vi "updateBall.vi"(8 "error in (no error)":errorcluster, 10 "old Ball":refnum<class "Ball.lvclass">, 11 "Ball in":refnum<class "Ball.lvclass">) -> (0 "error out":errorcluster, 3 "Ball out":refnum<class "Ball.lvclass">)   [LabVIEW 2020, in "Ball.lvclass"]
uses:
  Ball.lvclass
  C:/Users/Administrator/Desktop/SSL/SSL_AI/Object_class/Object.lvclass
  Object_class/Object.lvclass/Object.ctl
  Ball.lvclass/Ball.ctl
  Object_class/Read x.vi
  Object_class/Read y.vi
  Read v_x.vi
  Read v_y.vi
  Object_class/Read pos_est_x.vi
  Object_class/Read pos_est_y.vi
  Read Valid.vi
  Read z.vi
  Object_class/Write x.vi
  Object_class/Write y.vi
  Write v_x.vi
  Write v_y.vi
  Object_class/Write pos_est_x.vi
  Object_class/Write pos_est_y.vi
  Write Valid.vi
  Write z.vi
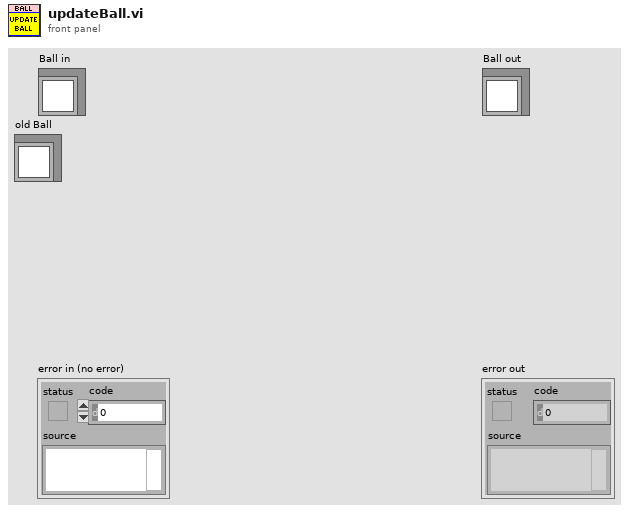
[diagram p1: front panel]
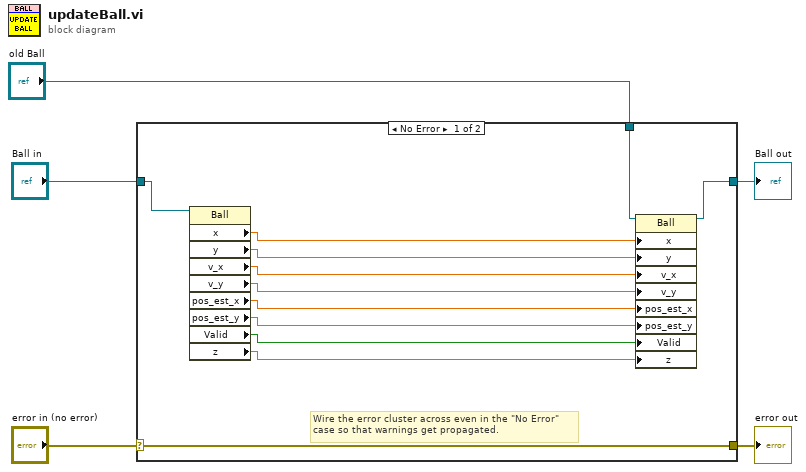
[diagram p0: block diagram]
diagram:
  n1 = case shown="No Error" "error in (no error)" {
    selector: "error in (no error)" -> [w17 w19]
    tunnel: [w17 w19] -> w4
    tunnel: [w15 w18] -> w2
    tunnel: "Ball in" -> [w16 w18]
    tunnel: "old Ball" -> [w14 _]
    frame No Error {
      # "Wire the error cluster across even in the \"No Error\"\ncase so that warnings get propagated."
      n2 = property class="Ball"(reference=w16) -> ("x"=w13:dbl, "y"=w12:dbl, "v_x"=w11:dbl, "v_y"=w10:dbl, "pos_est_x"=w9:dbl, "pos_est_y"=w8:dbl, "Valid"=w7:bool, "z"=w6:dbl)  [unwired: 1 in, 2 out]
      n3 = property class="Ball"(reference=w14, "x"=w13, "y"=w12, "v_x"=w11, "v_y"=w10, "pos_est_x"=w9, "pos_est_y"=w8, "Valid"=w7, "z"=w6) -> (reference out=w15:refnum<class "Ball.lvclass">)  [unwired: 1 in, 1 out]
    }
    frame Error {
    }
  }
  "error out" <- w4
  "Ball out" <- w2
